vi "04Foot.vi"() -> ()   [LabVIEW 2020]
uses:
  <vilib>/DAQmx/read.llb/DAQmx Read (Digital 1D U8 1Chan NSamp).vi
  <vilib>/Instr/_visa.llb/VISA Configure Serial Port (Serial Instr).vi
  <vilib>/Utility/file.llb/Read Delimited Spreadsheet (DBL).vi
  <vilib>/DAQmx/create/channels.llb/DAQmx Create Channel (DI-Digital Input).vi
  <vilib>/DAQmx/configure/timing.llb/DAQmx Timing (Change Detection).vi
  <vilib>/DAQmx/miscellaneous.llb/DAQmx Fill In Error Info.vi
panel:
  out "MPH READ 2":u8
  in  "Tab Control":enum32{"Page 1", "Page 2", "Page 3"}(tab)
  out "NEXT INC":dbl min=0.0 max=12.0 step=0.1 format="%.1f"
  out "INC":dbl min=0.0 max=12.0 step=0.1 format="%.1f"
  out "NEXT DURATION":dbl format="%#.1f"
  out "NEXT MPH":dbl min=0.0 max=12.0 step=0.1 format="%.1f"
  out "Time Left":dbl format="%#.0f"
  out "ESTOP":bool
  in  "ESTOP RESUME":bool
  out "MPH":dbl min=0.0 max=12.0 step=0.1 format="%.1f"
  out "incline":dbl[](array[numeric])
  out "ESTOP2":bool
  out "Report Location":path
  in  "TestScript":path=path "C:/LabView Computer Backup SEAL2788/DonP_TRM500/FootTimeInc.txt"
  out "Waveform Graph":dbl[](graph)
  out "speed":dbl[](array[numeric])
  out "time":dbl[](array[numeric])
  out "dwell":dbl[](array[numeric])
  out "step":i32
  out "arraysize":i32
  out "x-y":u32
  out "appended path":path
  out "stopping":bool
  out "String":string
  in  "stop":bool
  out "MPH READ":u8
  in  "Serial Port":refnum<visa-resource-name>="COM8"
  in  "lines":tag="cDAQ1Mod1/port0/line0"
  out "Enum":T1(ring)
  out "FootPath":path
  out "Array":T2(array[cluster])
  out "size(s)":i32
  out "FootPathRef":refnum<file>
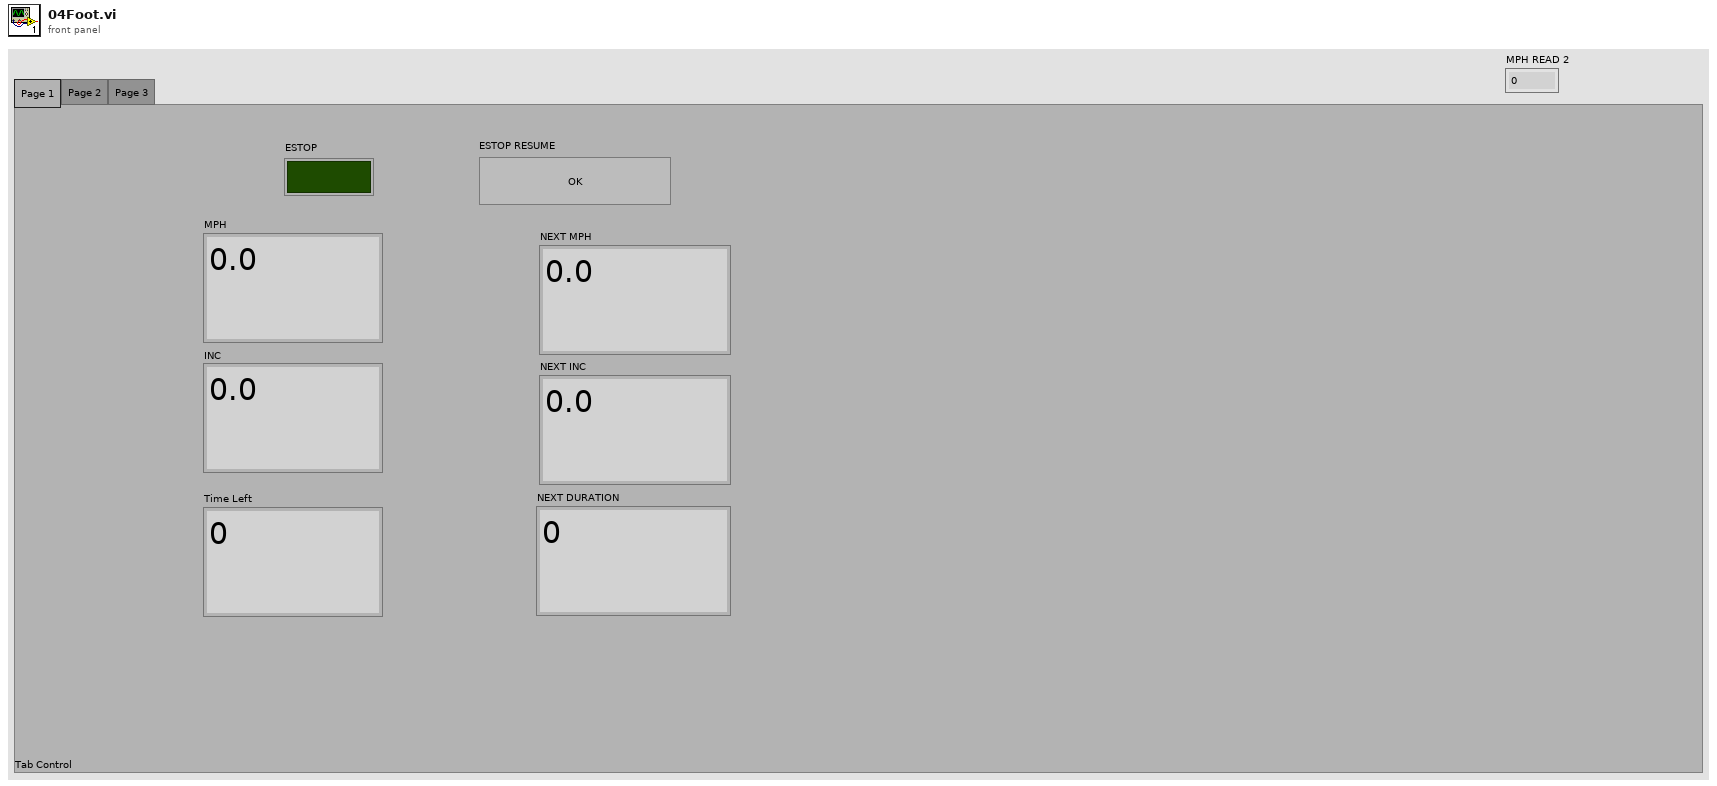
[diagram p1: front panel]
types:
  T1 = enum16{"Initialize", "SetMPH", "GetData", "CheckTiming", "CompressWave", "StartDAQ", "StopDAQ", "Dwell", "WaitforMPH", "ESTOP Wait", "ESTOP Resume"}
  T2 = cluster{"Trigger Time":timestamp, "MPH":dbl, "INC":dbl}[]
  T3 = cluster{"seconds since 1Jan1904":timestamp, "MPH":dbl, "INC":dbl}[]
  T4 = cluster{"Time":timestamp, "MPH":dbl, "INC":dbl}[]
  T5 = enum16{"Initialize", "SetMPH", "GetData", "CheckTiming", "CompressWave", "StartDAQ"}
  T6 = enum16{"Initialize", "SetMPH", "GetData", "CheckTiming", "CompressWave", "StartDAQ", "StopDAQ"}
  T7 = enum16{"Initialize", "SetMPH", "GetData", "CheckTiming", "CompressWave", "StartDAQ", "StopDAQ", "Dwell", "WaitforMPH"}
  T8 = cluster{"seconds since 1Jan1904":timestamp, "MPH":dbl, "INC":dbl}
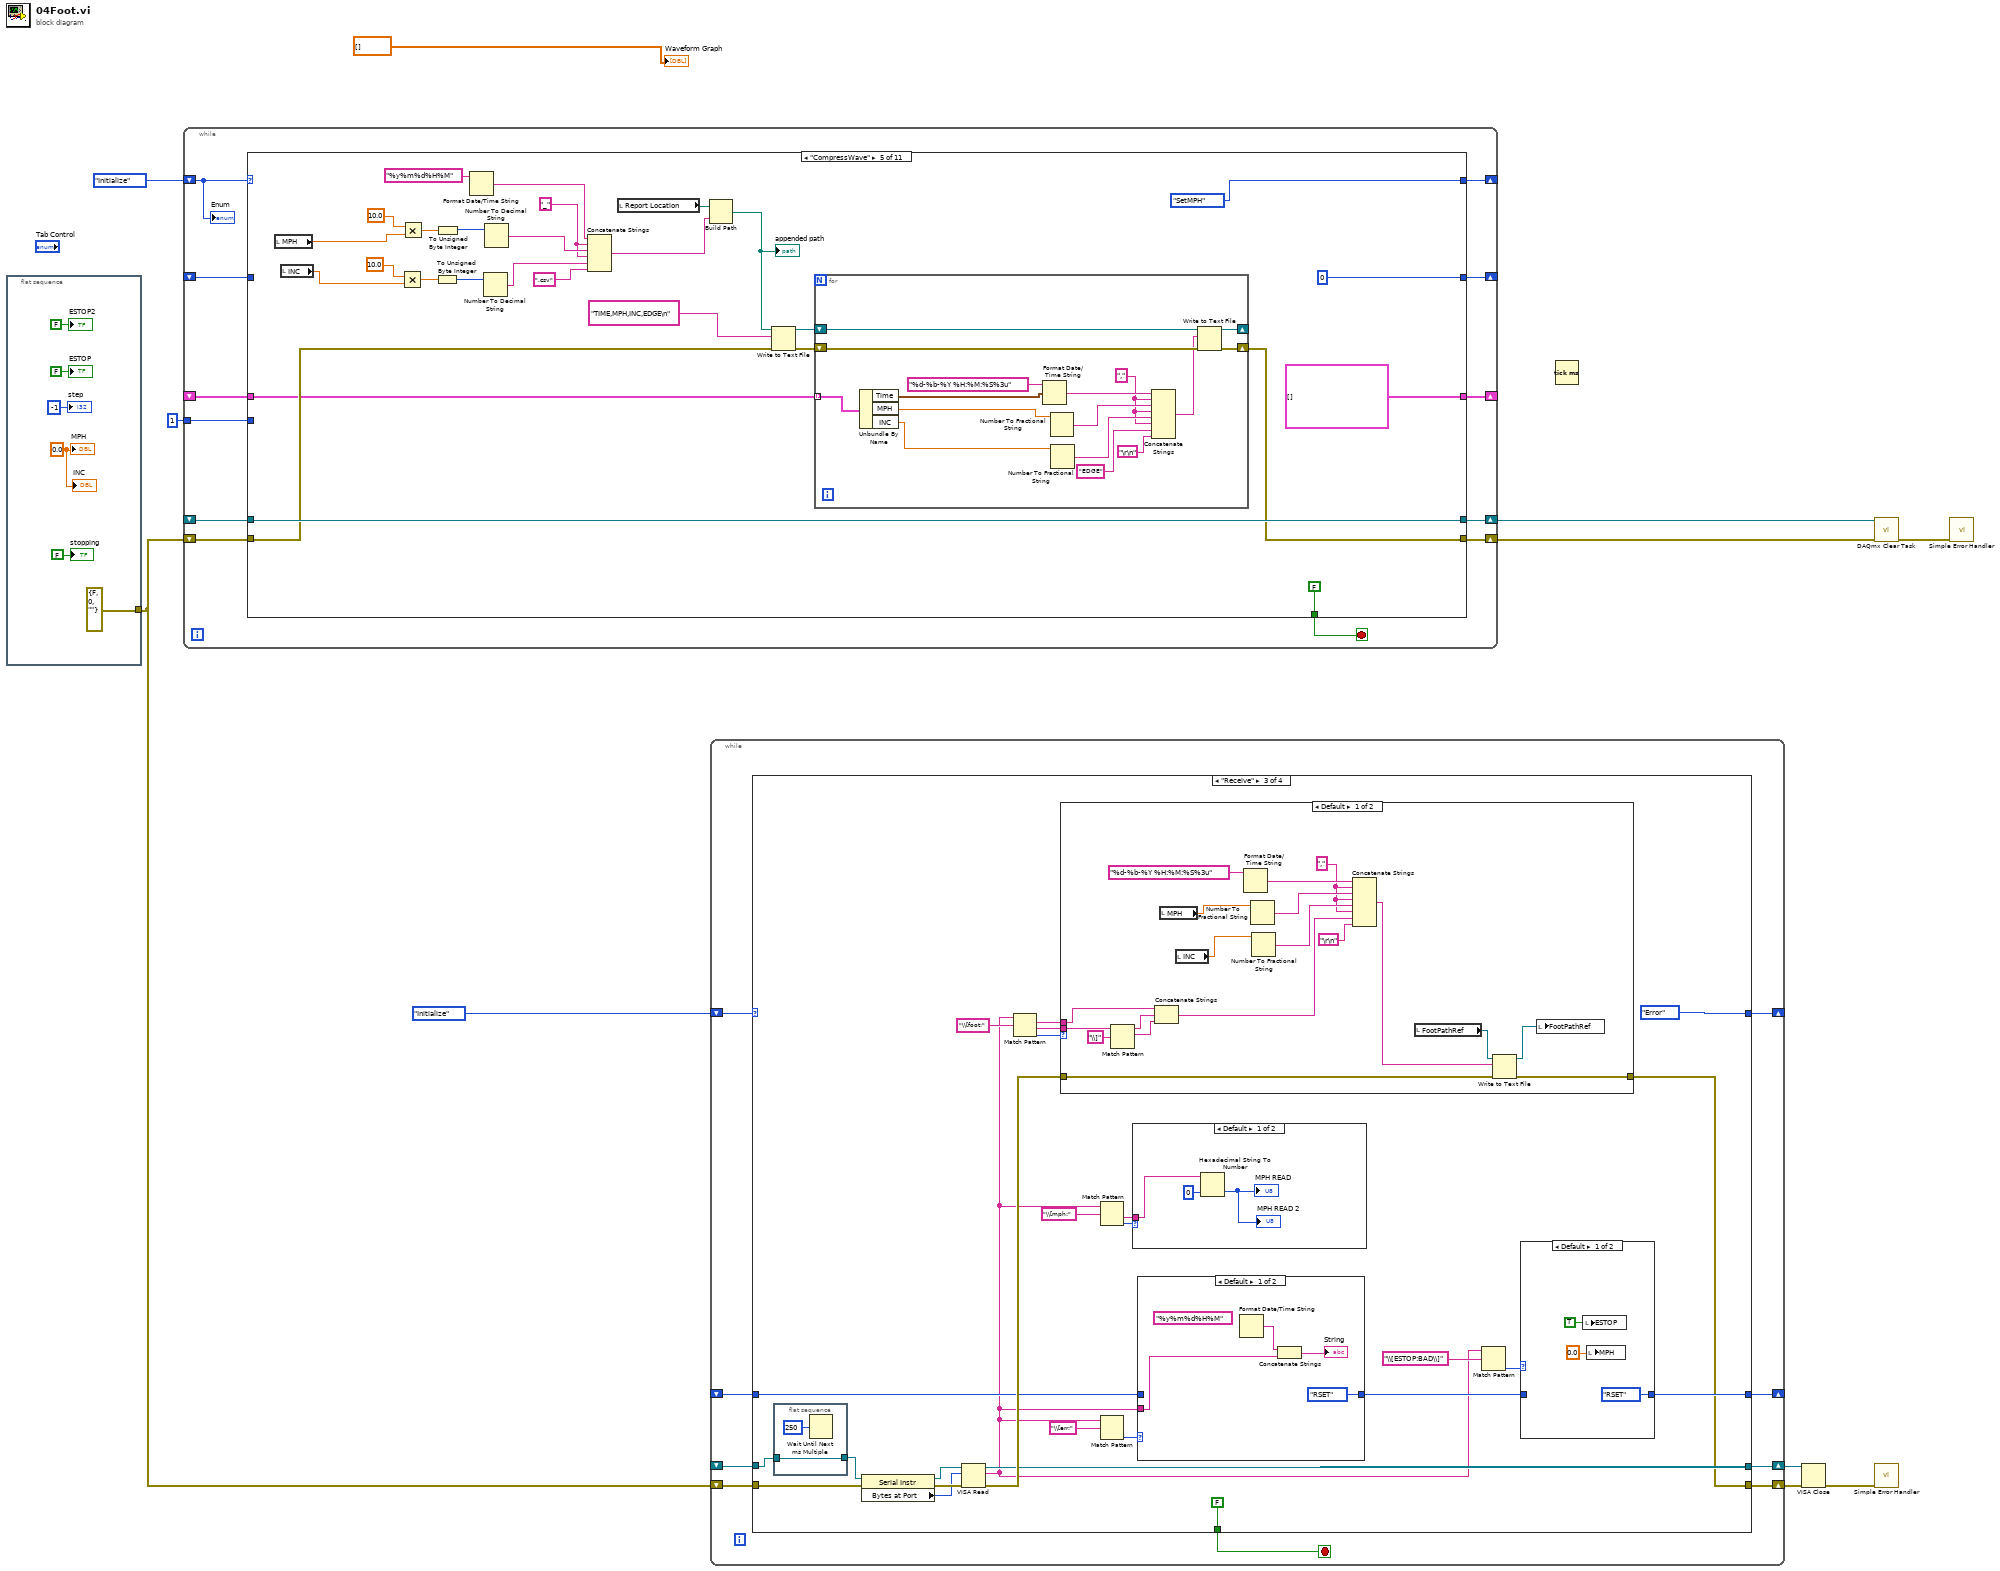
[diagram p0: block diagram]
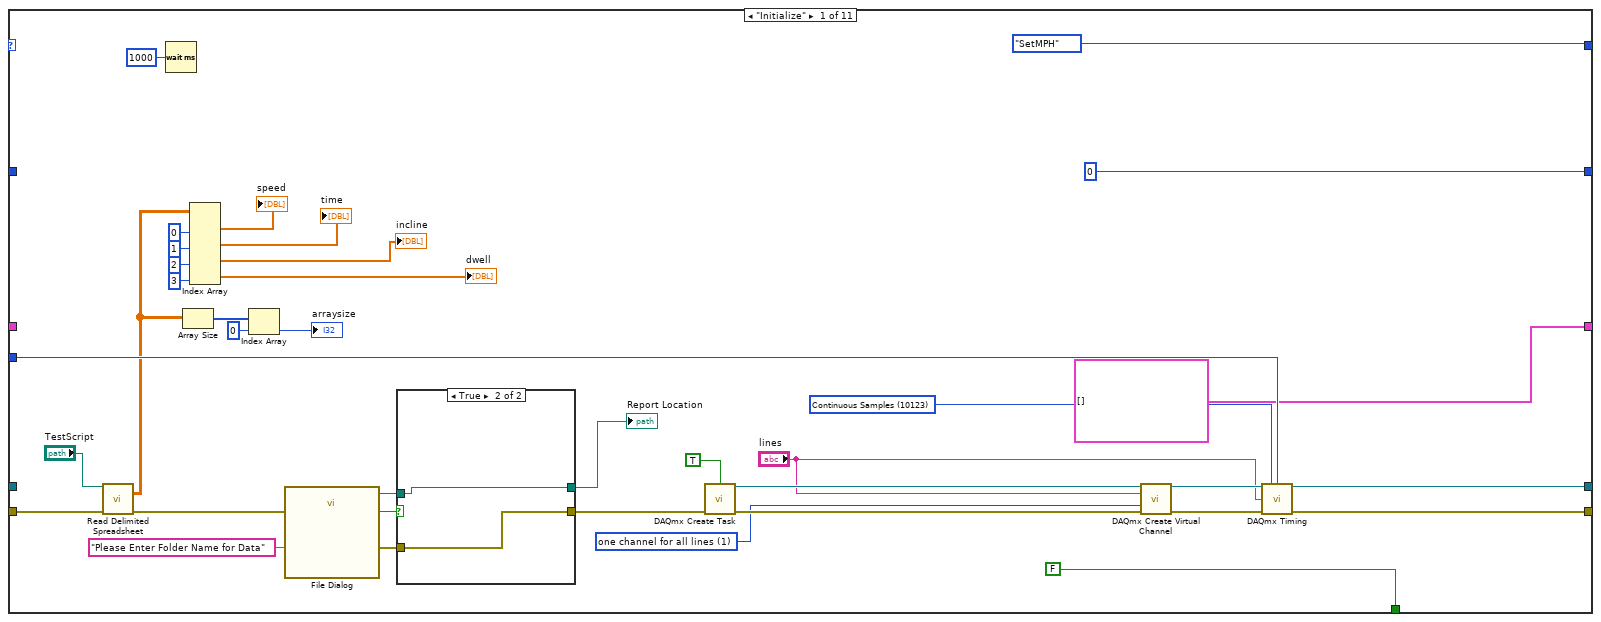
[diagram p2: hidden frame]
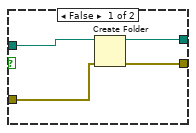
[diagram p3: hidden frame]
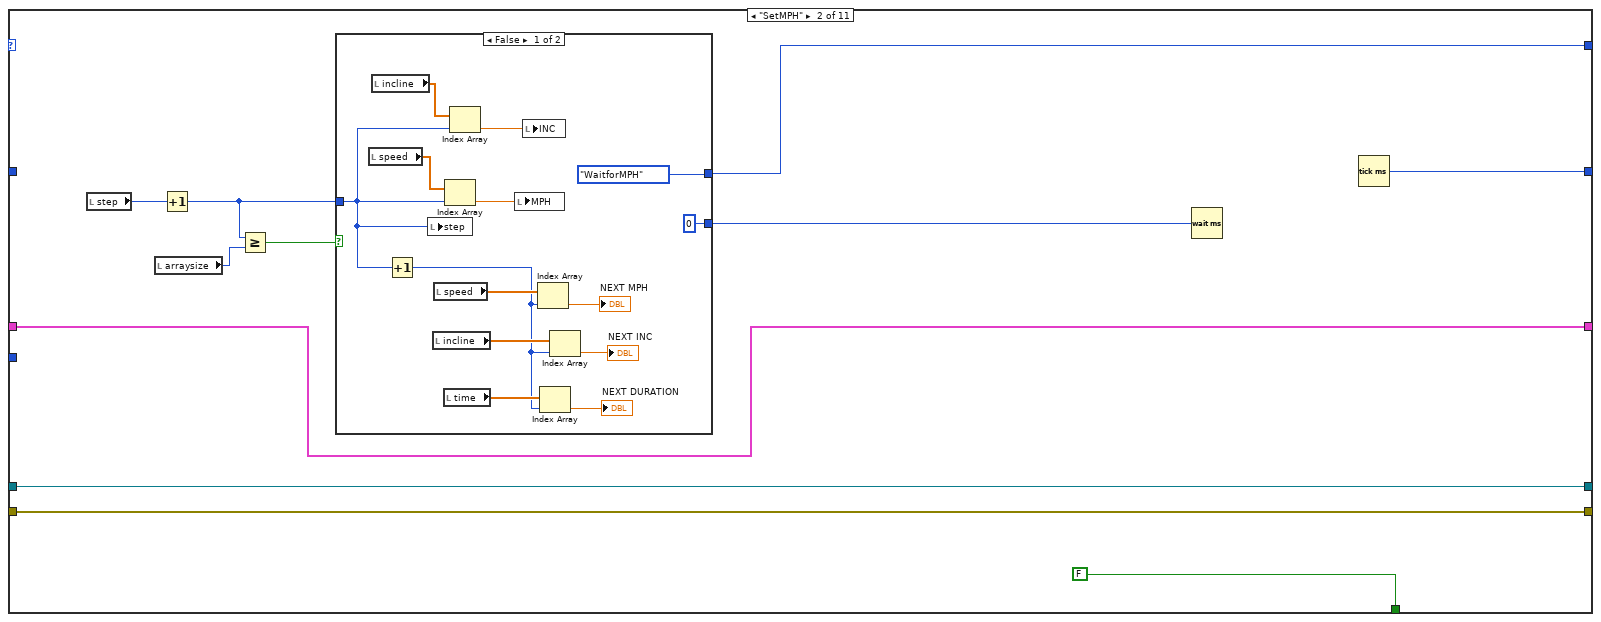
[diagram p4: hidden frame]
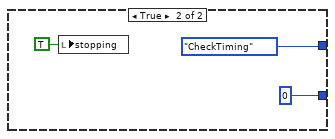
[diagram p5: hidden frame]
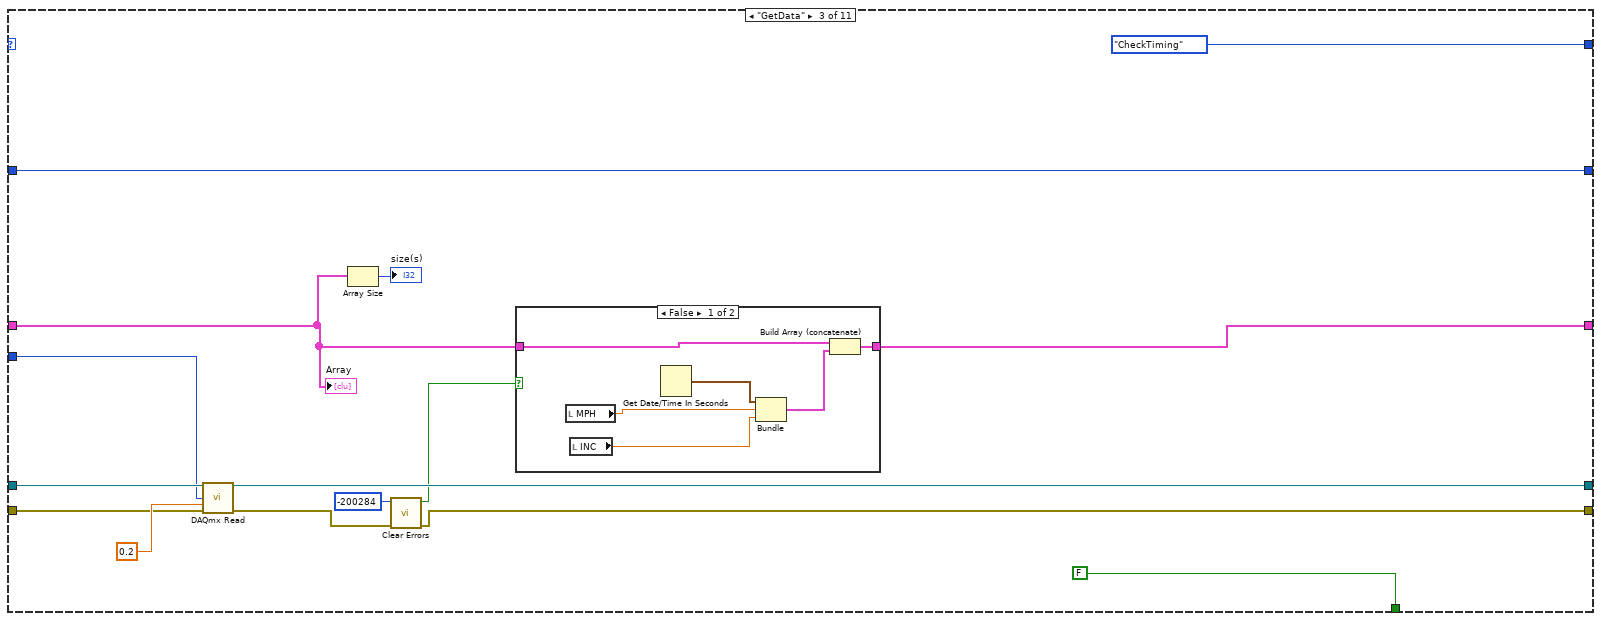
[diagram p6: hidden frame]
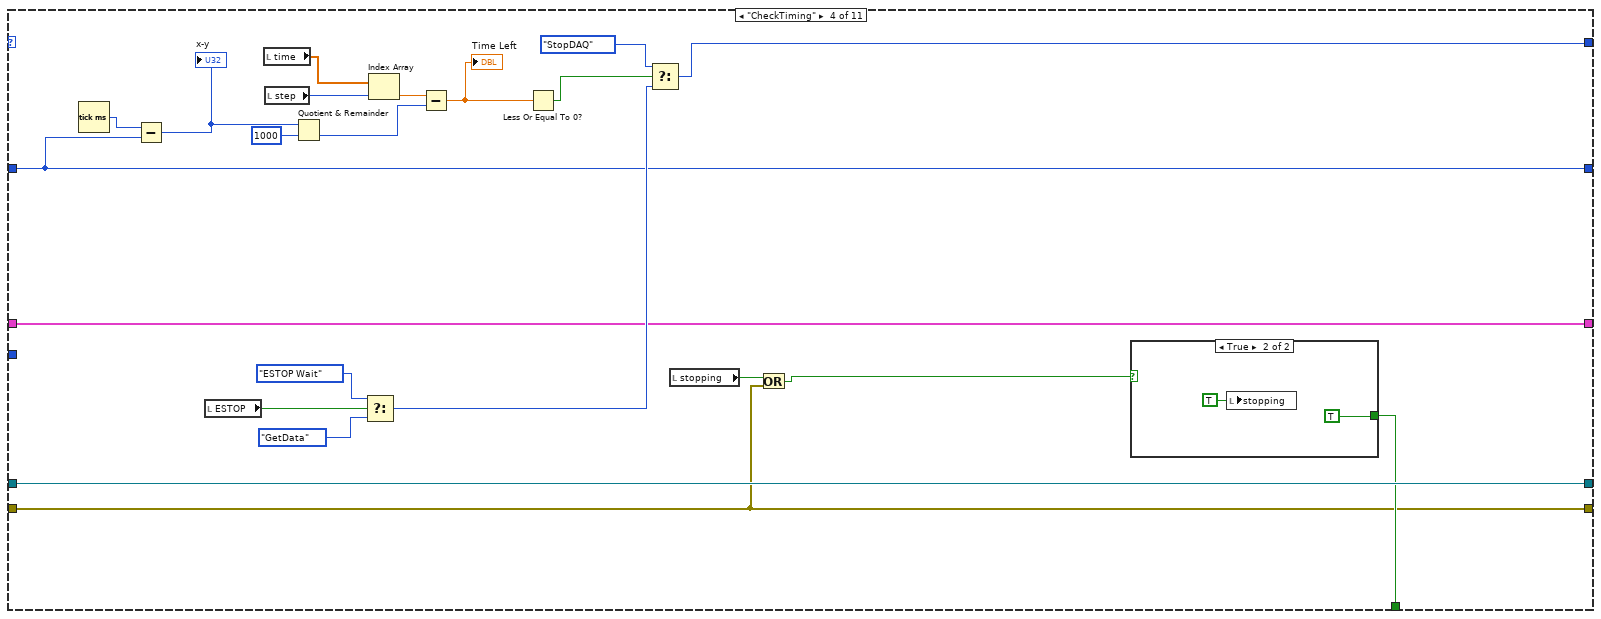
[diagram p8: hidden frame]
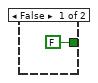
[diagram p9: hidden frame]
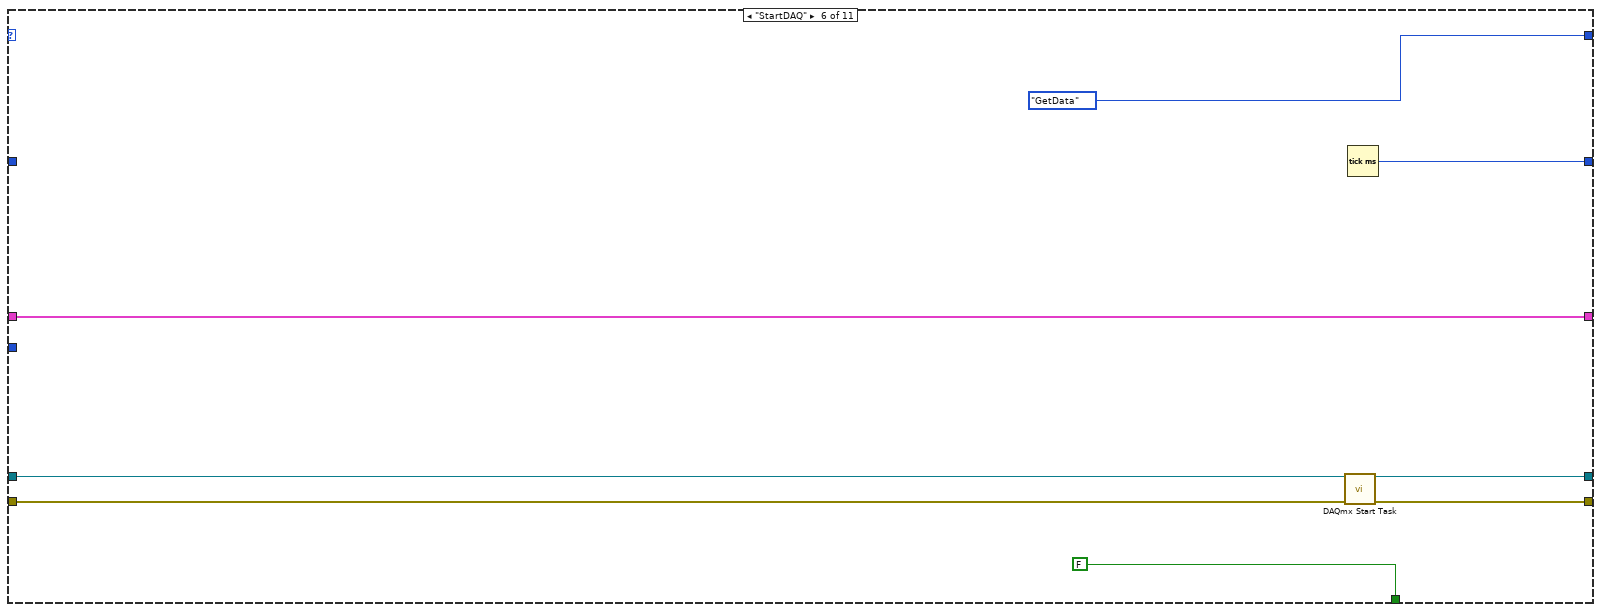
[diagram p10: hidden frame]
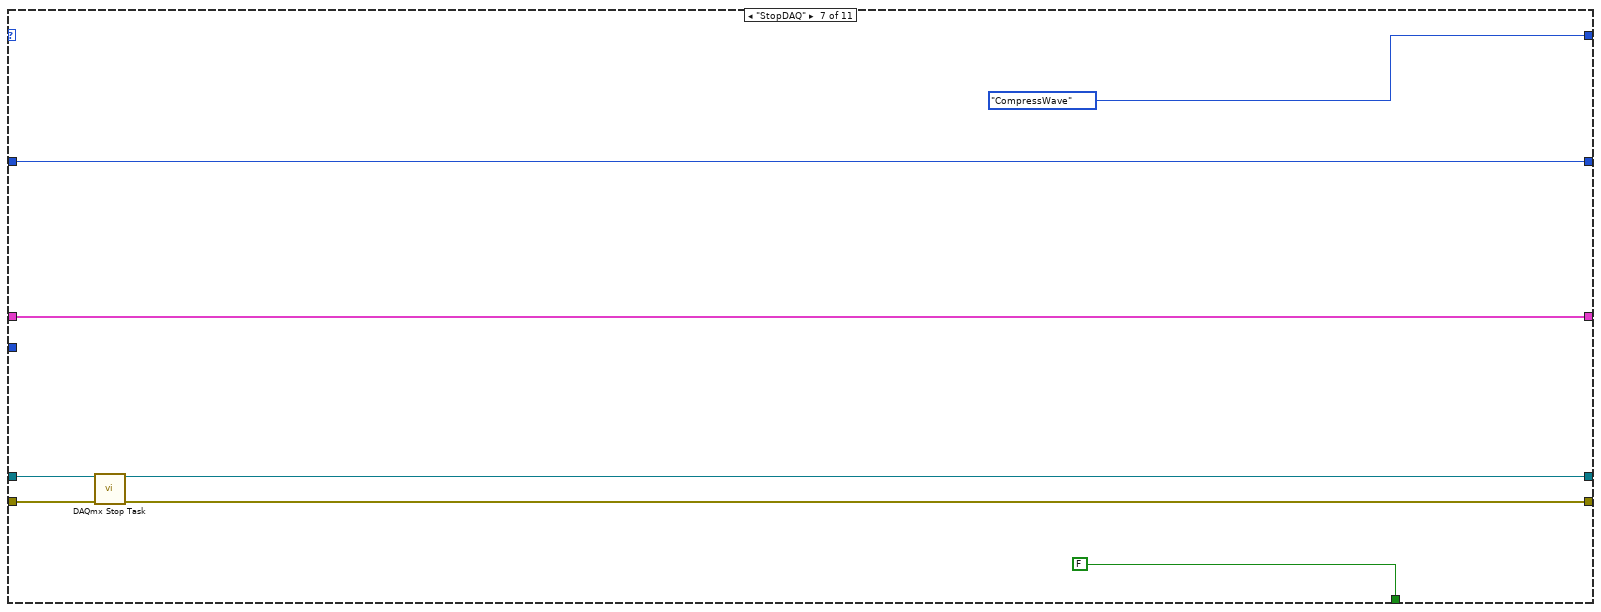
[diagram p11: hidden frame]
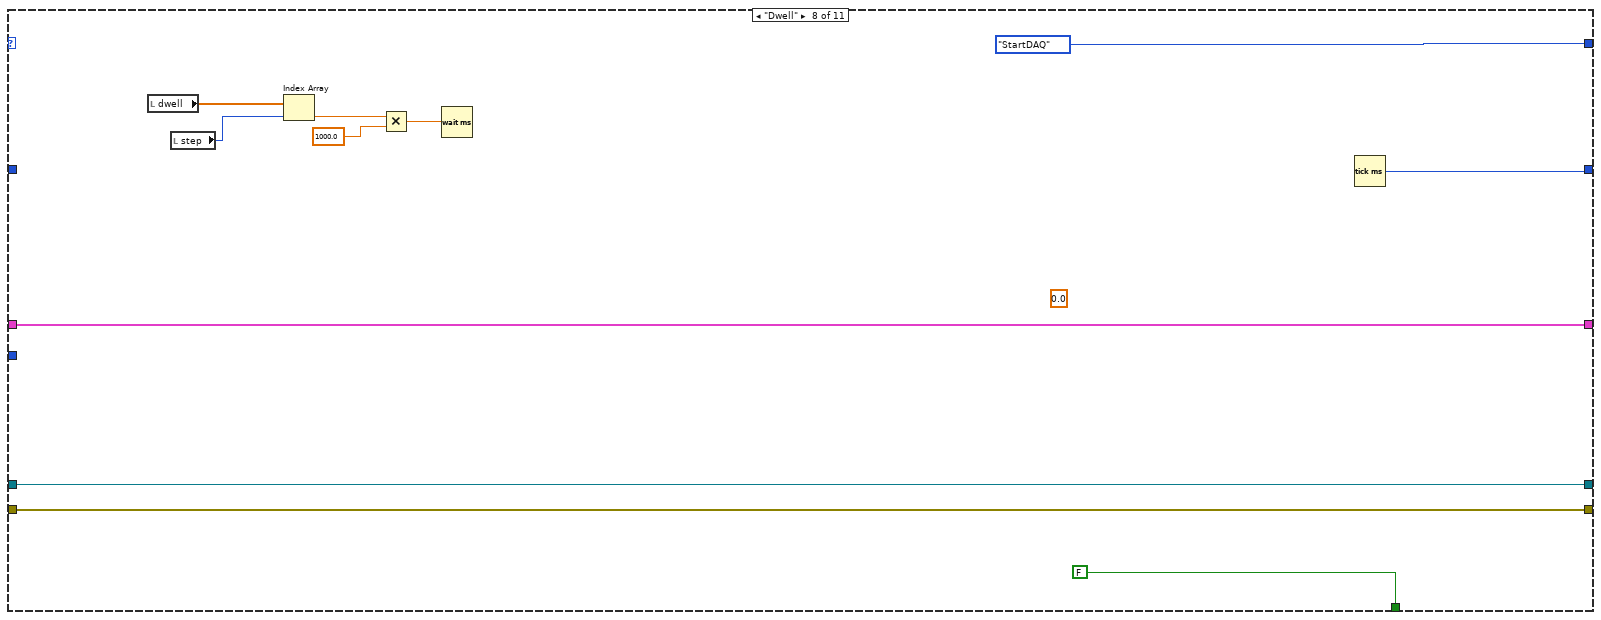
[diagram p12: hidden frame]
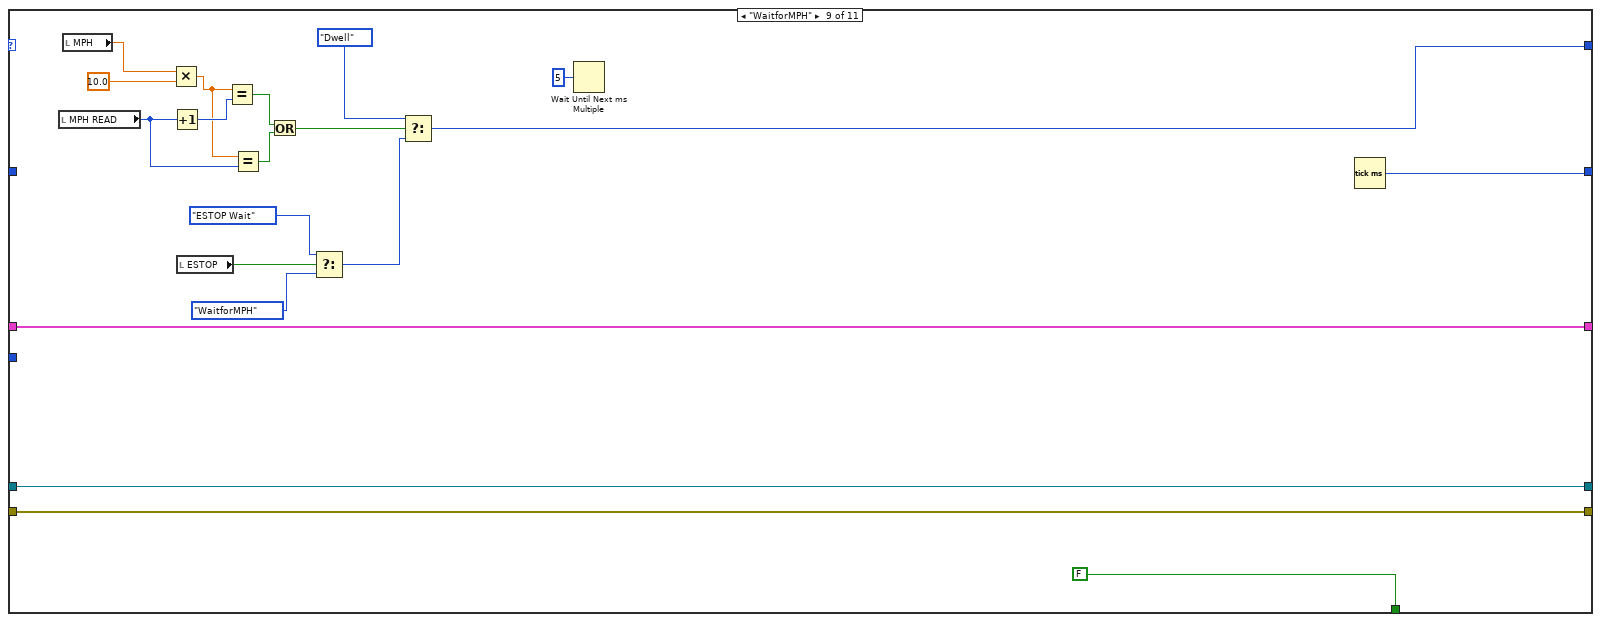
[diagram p13: hidden frame]
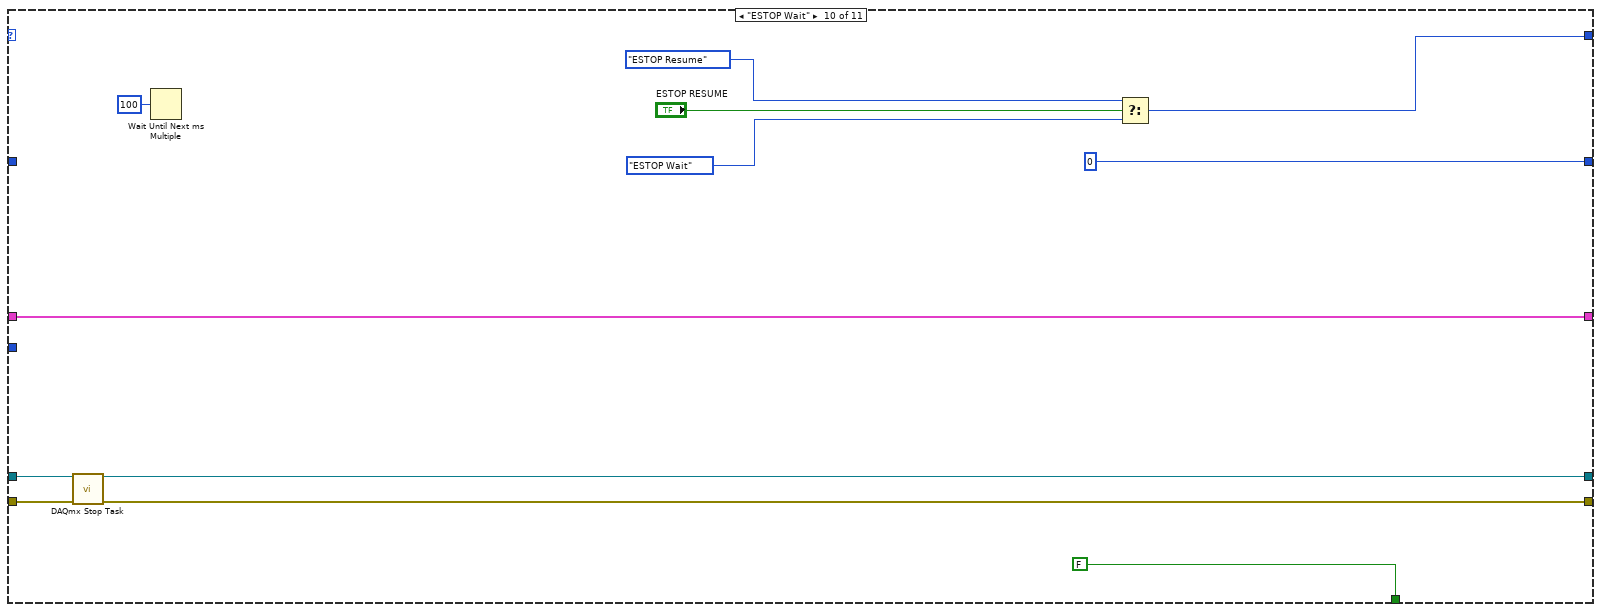
[diagram p14: hidden frame]
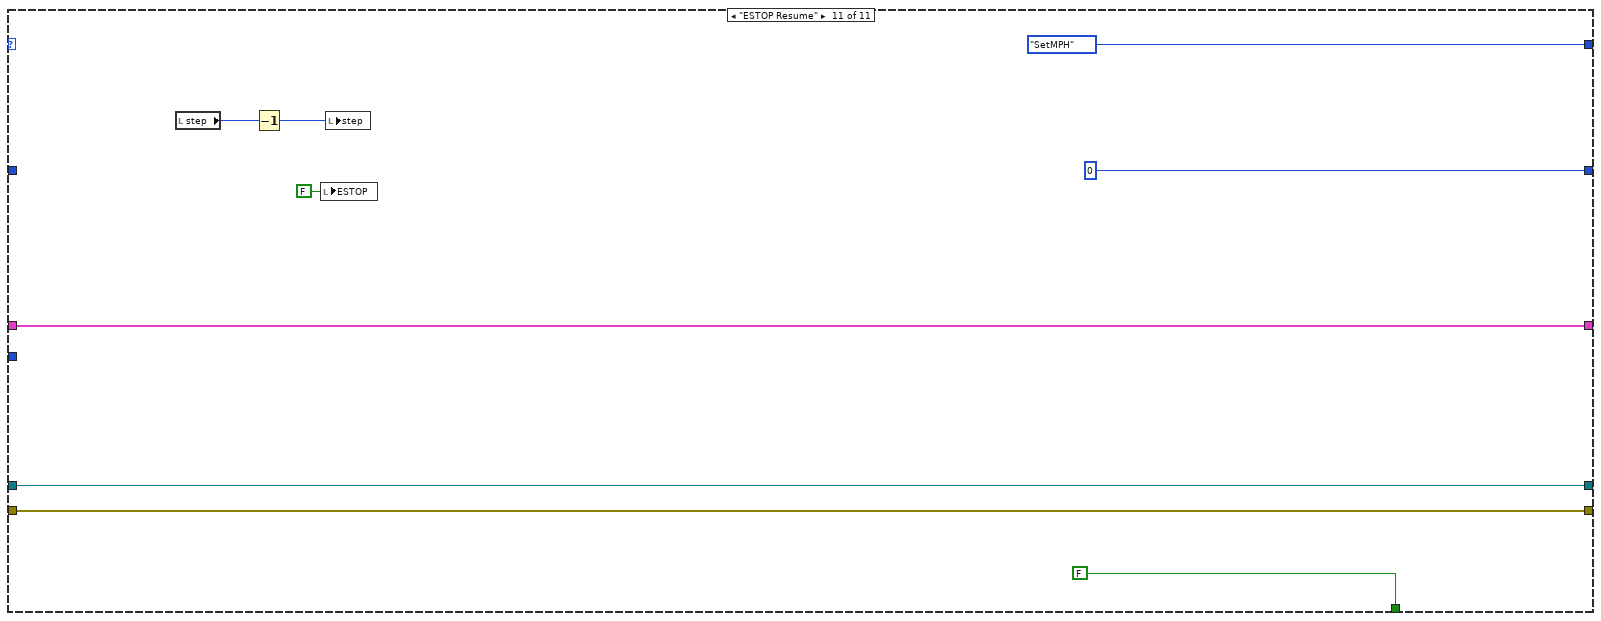
[diagram p15: hidden frame]
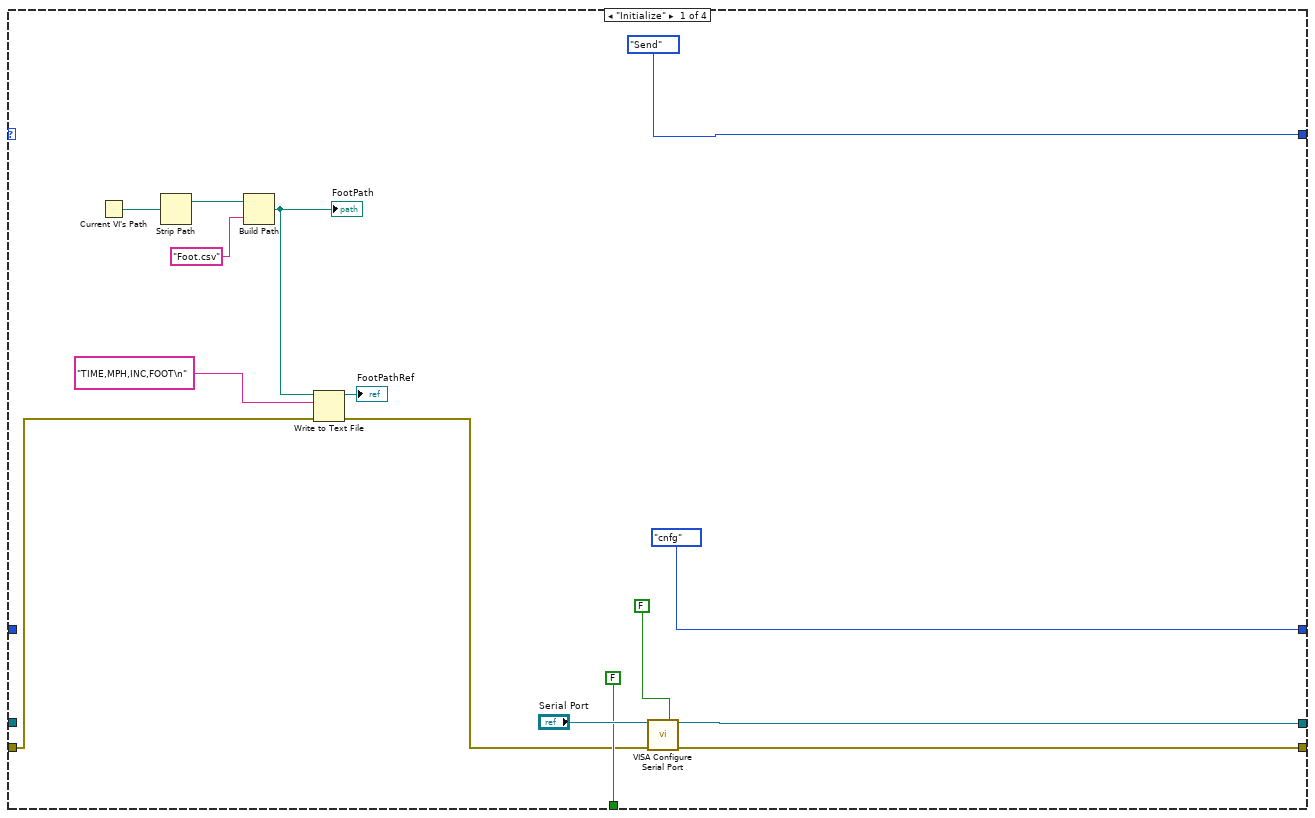
[diagram p16: hidden frame]
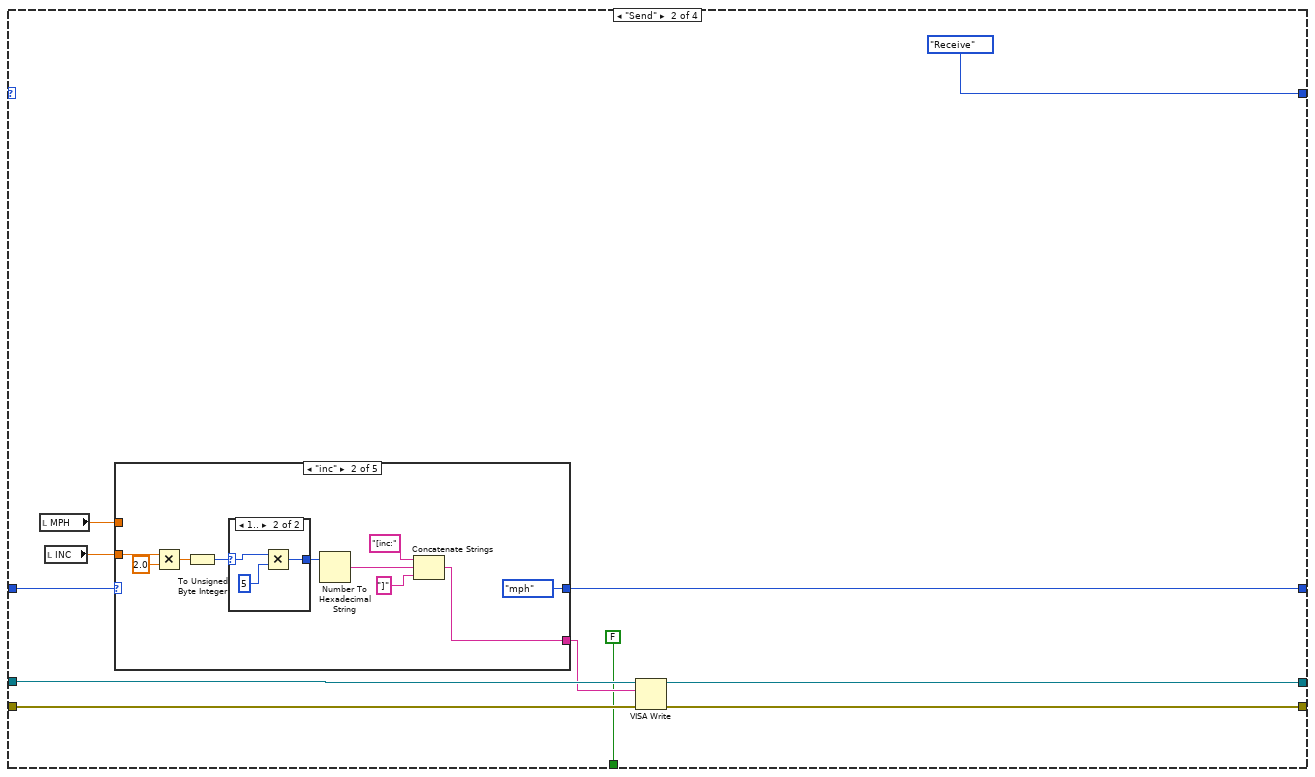
[diagram p17: hidden frame]
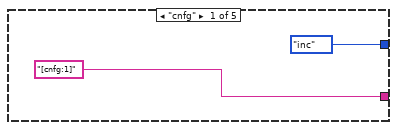
[diagram p18: hidden frame]
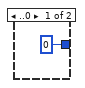
[diagram p19: hidden frame]
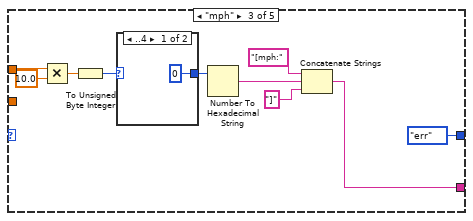
[diagram p20: hidden frame]
diagram:
  n1 = flat-sequence {
    tunnel: [errorcluster {"status"=FALSE, "code"=0, "source"=""} ("error constant")] -> w3
    frame #0 {
      w12 = 0.0 ("MPH")
      "stopping" <- FALSE ("stopping")
      "MPH" <- w12
      "step" <- -1 ("step")
      "ESTOP" <- FALSE ("ESTOP")
      "ESTOP2" <- FALSE ("ESTOP2")
      "INC" <- w12
    }
  }
  n2 = while {
    shift-right: [w29] -> _
    shift-left: T1."Initialize" -> [w20]
    shift-right: [w27] -> w5
    shift-left: _ -> [w25]
    shift-right: [w26] -> w6
    shift-left: w3 -> [w24]
    shift-right: [w23] -> _
    shift-left: _ -> [w22]
    tunnel: 1 ("samples per channel") -> [w21]
    shift-right: [w18] -> _
    shift-left: _ -> [w19]
    stop <- w28 stop-if-true
    n3 = case shown="\"CompressWave\"" w20 {
      tunnel: [T1."SetMPH" w79 T1."CheckTiming" ("f") w139 T1."SetMPH" T5."GetData" T6."CompressWave" T7."StartDAQ" w231 w245 T1."SetMPH" ("f")] -> w29
      tunnel: [FALSE FALSE FALSE w143 FALSE FALSE FALSE FALSE FALSE FALSE FALSE] -> w28
      tunnel: [w35 w81 w107 w144 w166 w196 w204 w217 w237 w241 w254] -> w27
      tunnel: [w36 w80 w106 w140 w148 w197 w203 w216 w236 w240 w255] -> w26
      tunnel: w25 -> [_ w81 w110 w144 w166 w195 w206 w217 w237 w243 w254]
      tunnel: w24 -> [w60 w80 w109 w140 w152 w194 w205 w216 w236 w242 w255]
      tunnel: [u32 0 w73 w114 w127 u32 0 w192 w201 w218 w238 u32 0 ("millisecond timer value") u32 0 ("millisecond timer value")] -> w23
      tunnel: w22 -> [_ _ w114 w127 _ _ w201 _ _ _ _]
      tunnel: w21 -> [w57 _ w108 _ _ _ _ _ _ _ _]
      tunnel: w19 -> [_ w74 w102 w126 w151 w193 w200 w208 w219 w239 w251]
      tunnel: [T3 [] w74 w105 w126 T4 [] w193 w200 w208 w219 w239 w251] -> w18
      frame "Initialize" {
        w56 = 10123 items=["Finite Samples"=10178, "Continuous Samples"=10123, "Hardware Timed Single Point"=12522] ("sample mode")
        w64 = 1 items=["one channel for each line", "one channel for all lines"] ("line grouping")
        n4 = call-poly <vilib>:"Read Delimited Spreadsheet.vi"("file path (dialog if empty)"="TestScript", "error in (no error)"=w60) -> ("all rows"=w47:dbl[][], "error out"=w45:errorcluster)  [unwired: 8 in, 4 out]
        n5 = Wait (ms)(milliseconds to wait=u32 1000) -> ()  [unwired: 1 out]
        n6 = Array Size(array=w47) -> (size(s)=w50:i32[])
        n7 = Index Array(array=w47, index (col) #1=0 ("disabled index (col)"), index (col) #2=1 ("index (col)"), index (col) #3=2 ("index (col)"), index (col) #4=3 ("index (col)")) -> (element #1=→"speed":dbl[], element #2=→"time":dbl[], element #3=→"incline":dbl[], element #4=→"dwell":dbl[])  [unwired: 4 in]
        n8 = Index Array(array=w50, index=0) -> (element=→"arraysize":i32)
        n9 = call "File Dialog"("prompt"="Please Enter Folder Name for Data", "error in"=w45) -> ("selected path"=w41:path, "exists"=w43:bool, "error out"=w42:errorcluster)  [unwired: 10 in, 1 out]
        n10 = case shown="True" w43 {
          tunnel: w42 -> [w70 w71]
          tunnel: w41 -> [w69 w72]
          tunnel: [w68 w71] -> w40
          tunnel: [w67 w72] -> w39
          frame False {
            n11 = Create Folder(path (use dialog)=w69, error in=w70) -> (created path=w67:path, error out=w68:errorcluster)  [unwired: 1 in, 1 out]
          }
          frame True {
          }
        }
        "Report Location" <- w39
        n12 = call <vilib>:"DAQmx Create Task.vi"("auto cleanup"=TRUE, "error in"=w40) -> ("task out"=w66:refnum<k21>, "error out"=w65:errorcluster)  [unwired: 12 in]
        n13 = call-poly <vilib>:"DAQmx Create Virtual Channel.vi"("task in"=w66, "lines"="lines", "line grouping"=w64, "error in"=w65) -> ("task out"=w58:refnum<k21>, "error out"=w59:errorcluster)  [unwired: 10 in]
        n14 = call-poly <vilib>:"DAQmx Timing.vi"("task/channels in"=w58, "sample mode"=w56, "samples per channel"=w57, "rising edge physical channels"="lines", "error in"=w59) -> ("task out"=w35:refnum<k21>, "error out"=w36:errorcluster)  [unwired: 9 in]
      }
      frame "SetMPH" {
        n15 = local read "step"() -> (w76:i32)
        n16 = local read "arraysize"() -> (w78:i32)
        n17 = Increment(x=w76) -> (x+1=w75:i32)
        n18 = Greater Or Equal?(x=w75, y=w78) -> (x >= y?=w77:bool)
        n19 = case shown="False" w77 {
          tunnel: [u32 0 ("milliseconds to wait") u32 0 ("milliseconds to wait")] -> w82
          tunnel: [T1."WaitforMPH" T1."CheckTiming"] -> w79
          tunnel: w75 -> [w86 _]
          frame False {
            n20 = local read "speed"() -> (w96:dbl[])
            n21 = local read "incline"() -> (w87:dbl[])
            n22 = Increment(x=w86) -> (x+1=w88:i32)
            n23 = local write "step"(w86) -> ()
            n24 = local read "incline"() -> (w89:dbl[])
            n25 = local read "speed"() -> (w94:dbl[])
            n26 = local read "time"() -> (w91:dbl[])
            n27 = Index Array(array=w96, index=w86) -> (element=w95:dbl)
            n28 = Index Array(array=w87, index=w86) -> (element=w85:dbl)
            n29 = local write "MPH"(w95) -> ()
            n30 = local write "INC"(w85) -> ()
            n31 = Index Array(array=w94, index=w88) -> (element=→"NEXT MPH":dbl)
            n32 = Index Array(array=w91, index=w88) -> (element=→"NEXT DURATION":dbl)
            n33 = Index Array(array=w89, index=w88) -> (element=→"NEXT INC":dbl)
          }
          frame True {
            n34 = local write "stopping"(TRUE ("stopping")) -> ()
          }
        }
        n35 = Wait (ms)(milliseconds to wait=w82) -> ()  [unwired: 1 out]
        n36 = Tick Count (ms)() -> (millisecond timer value=w73:u32)
      }
      frame "GetData" {
        n37 = call-poly <vilib>:"DAQmx Read.vi"("task/channels in"=w110, "number of samples per channel"=w108, "timeout"=0.2, "error in"=w109) -> ("task out"=w107:refnum<k21>, "error out"=w111:errorcluster)  [unwired: 9 in, 1 out]
        n38 = Array Size(array=w102) -> (size(s)=→"size(s)":i32)
        n39 = call <vilib>:"Clear Errors.vi"("error in (no error)"=w111, "specific error code to clear (0: all)"=-200284) -> ("error out"=w106:errorcluster, "specific error cleared?"=w103:bool)  [unwired: 4 in]
        n40 = case shown="False" w103 {
          tunnel: [w121 w122] -> w105
          tunnel: w102 -> [w120 w122]
          frame False {
            n41 = local read "MPH"() -> (w117:dbl)
            n42 = local read "INC"() -> (w116:dbl)
            n43 = Get Date/Time In Seconds() -> (seconds since 1Jan1904=w119:timestamp)
            n44 = Bundle("seconds since 1Jan1904"=w119, "MPH"=w117, "INC"=w116) -> (w118:T8)  [unwired: 1 in]
            n45 = Build Array (concatenate)(w120, w118) -> (w121:T3)
          }
          frame True {
          }
        }
        "Array" <- w102
      }
      frame "CheckTiming" {
        n46 = Tick Count (ms)() -> (millisecond timer value=w128:u32)
        n47 = Subtract(x=w128, y=w127) -> (x-y=w125:u32)
        "x-y" <- w125
        n48 = local read "ESTOP"() -> (w134:bool)
        n49 = local read "time"() -> (w138:dbl[])
        n50 = local read "step"() -> (w137:i32)
        n51 = Quotient & Remainder(x=w125, y=u32 1000) -> (floor(x/y)=w123:u32)  [unwired: 1 out]
        n52 = Select(t=T1."ESTOP Wait", s=w134, f=T1."GetData") -> (s? t:f=w132:T1)
        n53 = Index Array(array=w138, index=w137) -> (element=w131:dbl)
        n54 = Subtract(x=w131, y=w123) -> (x-y=w130:dbl)
        "Time Left" <- w130
        n55 = Less Or Equal To 0?(x=w130) -> (x <= 0?=w129:bool)
        n56 = Select(t=T1."StopDAQ", s=w129, f=w132) -> (s? t:f=w139:T1)
        n57 = local read "stopping"() -> (w142:bool)
        n58 = Or(x=w142, y=w140) -> (x .or. y?=w141:bool)
        n59 = case shown="True" w141 {
          tunnel: [FALSE TRUE] -> w143
          frame False {
          }
          frame True {
            n60 = local write "stopping"(TRUE ("stopping")) -> ()
          }
        }
      }
      frame "CompressWave" {
        w160 = "_" ("string")
        n61 = local read "MPH"() -> (w167:dbl)
        n62 = local read "INC"() -> (w156:dbl)
        n63 = Multiply(x=10.0, y=w156) -> (x*y=w158:dbl)
        n64 = Multiply(x=10.0, y=w167) -> (x*y=w170:dbl)
        n65 = To Unsigned Byte Integer(number=w158) -> (unsigned 8bit integer=w157:u8)
        n66 = To Unsigned Byte Integer(number=w170) -> (unsigned 8bit integer=w169:u8)
        n67 = Format Date/Time String(time format string (%c)="%y%m%d%H%M") -> (date/time string=w163:string)  [unwired: 2 in]
        n68 = Number To Decimal String(number=w157) -> (decimal integer string=w155:string)  [unwired: 1 in]
        n69 = Number To Decimal String(number=w169) -> (decimal integer string=w168:string)  [unwired: 1 in]
        n70 = Concatenate Strings(w163, w160, w168, w160, w155, ".csv" ("string")) -> (w172:string)
        n71 = local read "Report Location"() -> (w165:path)
        n72 = Build Path(base path=w165, name or relative path=w172) -> (appended path=w153:path)
        "appended path" <- w153
        n73 = Write to Text File(file (use dialog)=w153, text="TIME,MPH,INC,EDGE\n", error in=w152) -> (refnum out=w150:refnum<file>, error out=w149:errorcluster)  [unwired: 1 in, 1 out]
        n74 = for {
          tunnel: w151 -> [w191] mode=indexing
          shift-right: [w177] -> _
          shift-left: w150 -> [w180]
          shift-right: [w176] -> w148
          shift-left: w149 -> [w179]
          w185 = ","
          n75 = Unbundle By Name(w191) -> ("Time"=w183:timestamp, "MPH"=w182:dbl, "INC"=w181:dbl)
          n76 = Format Date/Time String(time format string (%c)="%d-%b-%Y %H:%M:%S%3u", seconds (now)=w183) -> (date/time string=w189:string)  [unwired: 1 in]
          n77 = Number To Fractional String(number=w182) -> (F-format string=w188:string)  [unwired: 3 in]
          n78 = Number To Fractional String(number=w181) -> (F-format string=w187:string)  [unwired: 3 in]
          n79 = Concatenate Strings(w189, w185, w188, w185, w187, w185, "EDGE", "\r\n") -> (w178:string)
          n80 = Write to Text File(file (use dialog)=w180, text=w178, error in=w179) -> (refnum out=w177:refnum<file>, error out=w176:errorcluster)  [unwired: 1 in, 1 out]
        }
      }
      frame "StartDAQ" {
        n81 = call <vilib>:"DAQmx Start Task.vi"("task/channels in"=w195, "error in"=w194) -> ("task out"=w196:refnum<k21>, "error out"=w197:errorcluster)  [unwired: 12 in]
        n82 = Tick Count (ms)() -> (millisecond timer value=w192:u32)
      }
      frame "StopDAQ" {
        n83 = call <vilib>:"DAQmx Stop Task.vi"("task/channels in"=w206, "error in"=w205) -> ("task out"=w204:refnum<k21>, "error out"=w203:errorcluster)  [unwired: 12 in]
      }
      frame "Dwell" {
        (unwired) 0.0
        n84 = local read "dwell"() -> (w214:dbl[])
        n85 = local read "step"() -> (w213:i32)
        n86 = Index Array(array=w214, index=w213) -> (element=w212:dbl)
        n87 = Multiply(x=w212, y=1000.0) -> (x*y=w210:dbl)
        n88 = Wait (ms)(milliseconds to wait=w210) -> ()  [unwired: 1 out]
        n89 = Tick Count (ms)() -> (millisecond timer value=w218:u32)
      }
      frame "WaitforMPH" {
        n90 = local read "MPH READ"() -> (w223:u8)
        n91 = local read "MPH"() -> (w234:dbl)
        n92 = Multiply(x=w234, y=10.0) -> (x*y=w224:dbl)
        n93 = Increment(x=w223) -> (x+1=w232:u8)
        n94 = local read "ESTOP"() -> (w229:bool)
        n95 = Equal?(x=w224, y=w232) -> (x = y?=w221:bool)
        n96 = Equal?(x=w224, y=w223) -> (x = y?=w222:bool)
        n97 = Or(x=w221, y=w222) -> (x .or. y?=w220:bool)
        n98 = Select(t=T1."ESTOP Wait", s=w229, f=T1."WaitforMPH") -> (s? t:f=w226:T1)
        n99 = Select(t=T1."Dwell", s=w220, f=w226) -> (s? t:f=w231:T1)
        n100 = Wait Until Next ms Multiple(millisecond multiple=u32 5) -> ()  [unwired: 1 out]
        n101 = Tick Count (ms)() -> (millisecond timer value=w238:u32)
      }
      frame "ESTOP Wait" {
        n102 = call <vilib>:"DAQmx Stop Task.vi"("task/channels in"=w243, "error in"=w242) -> ("task out"=w241:refnum<k21>, "error out"=w240:errorcluster)  [unwired: 12 in]
        n103 = Wait Until Next ms Multiple(millisecond multiple=u32 100) -> ()  [unwired: 1 out]
        n104 = Select(t=T1."ESTOP Resume", s="ESTOP RESUME", f=T1."ESTOP Wait") -> (s? t:f=w245:T1)
      }
      frame "ESTOP Resume" {
        n105 = local read "step"() -> (w259:i32)
        n106 = Decrement(x=w259) -> (x-1=w258:i32)
        n107 = local write "ESTOP"(FALSE ("ESTOP")) -> ()
        n108 = local write "step"(w258) -> ()
      }
    }
    "Enum" <- w20
  }
  n109 = while {
    shift-right: [w264] -> w9
    shift-left: w3 -> [w268]
    shift-right: [w265] -> w10
    shift-left: _ -> [w267]
    shift-right: [w263] -> _
    shift-left: enum16{"Initialize", "Send", "Receive", "Error"}."Initialize" -> [w266]
    shift-right: [w262] -> _
    shift-left: _ -> [w261]
    stop <- w260 stop-if-true
    n110 = case shown="\"Receive\"" w266 {
      tunnel: w268 -> [w271 w292 w347 w388]
      tunnel: w267 -> [_ w291 w346 w392]
      tunnel: [w281 w294 w345 w392] -> w265
      tunnel: [w280 w293 w327 w388] -> w264
      tunnel: [enum16{"Initialize", "Send", "Receive", "Error"}."Send" enum16{"Initialize", "Send", "Receive", "Error"}."Receive" enum16{"Initialize", "Send", "Receive", "Error"}."Error" enum16{"Initialize", "Send", "Receive", "Error"}."Send"] -> w263
      tunnel: [enum16{"cnfg", "inc", "mph", "err", "RSET"}."cnfg" w288 w335 w393] -> w262
      tunnel: w261 -> [_ w289 w340 w393]
      tunnel: [FALSE FALSE FALSE w387] -> w260
      frame "Initialize" {
        n111 = Current VI's Path() -> (path=w276:path)
        n112 = Strip Path(path=w276) -> (stripped path=w275:path)  [unwired: 1 out]
        n113 = Build Path(base path=w275, name or relative path="Foot.csv") -> (appended path=w272:path)
        "FootPath" <- w272
        n114 = Write to Text File(file (use dialog)=w272, text="TIME,MPH,INC,FOOT\n", error in=w271) -> (refnum out=→"FootPathRef":refnum<file>, error out=w270:errorcluster)  [unwired: 1 in, 1 out]
        n115 = call-poly "VISA Configure Serial Port"("VISA resource name"="Serial Port", "Enable Termination\nChar (T)"=FALSE ("Enable Termination\nChar (T)"), "error in (no error)"=w270) -> ("VISA resource name out"=w281:refnum<visa-resource-name>, "error out"=w280:errorcluster)  [unwired: 11 in]
      }
      frame "Send" {
        n116 = local read "MPH"() -> (w285:dbl)
        n117 = local read "INC"() -> (w284:dbl)
        n118 = case shown="\"inc\"" w289 {
          tunnel: ["[cnfg:1]" w297 w311 "[err]" "[RSET]"] -> w290
          tunnel: w285 -> [_ _ w320 _ _]
          tunnel: [enum16{"cnfg", "inc", "mph", "err", "RSET"}."inc" enum16{"cnfg", "inc", "mph", "err", "RSET"}."mph" enum16{"cnfg", "inc", "mph", "err", "RSET"}."err" enum16{"cnfg", "inc", "mph", "err", "RSET"}."cnfg" enum16{"cnfg", "inc", "mph", "err", "RSET"}."cnfg"] -> w288
          tunnel: w284 -> [_ w298 _ _ _]
          frame "cnfg" {
          }
          frame "inc" {
            n119 = Multiply(x=w298, y=2.0) -> (x*y=w301:dbl)
            n120 = To Unsigned Byte Integer(number=w301) -> (unsigned 8bit integer=w300:u8)
            n121 = case shown="1.." w300 {
              selector: w300 -> [_ w310]
              tunnel: [u8 0 w309] -> w299
              frame ..0 {
              }
              frame 1.. {
                n122 = Multiply(x=w310, y=u8 5) -> (x*y=w309:u8)
              }
            }
            n123 = Number To Hexadecimal String(2:w299) -> (0:w304:string)  [unwired: 1 in]
            n124 = Concatenate Strings("[inc:" ("string"), w304, "]" ("string")) -> (w297:string)
          }
          frame "mph" {
            n125 = Multiply(x=w320, y=10.0) -> (x*y=w314:dbl)
            n126 = To Unsigned Byte Integer(number=w314) -> (unsigned 8bit integer=w313:u8)
            n127 = case shown="..4" w313 {
              selector: w313 -> [_ w322]
              tunnel: [u8 0 w322] -> w312
              frame ..4 {
              }
              frame 5.. {
              }
            }
            n128 = Number To Hexadecimal String(2:w312) -> (0:w317:string)  [unwired: 1 in]
            n129 = Concatenate Strings("[mph:" ("string"), w317, "]" ("string")) -> (w311:string)
          }
          frame "err" {
          }
          frame "RSET" {
          }
        }
        n130 = VISA Write(VISA resource name=w291, write buffer=w290, error in (no error)=w292) -> (VISA resource name out=w294:refnum<visa-resource-name>, error out=w293:errorcluster)  [unwired: 1 out]
      }
      frame "Receive" {
        n131 = flat-sequence {
          tunnel: w346 -> [w385]
          tunnel: [w385] -> w351
          frame #0 {
            n132 = Wait Until Next ms Multiple(millisecond multiple=u32 250) -> ()  [unwired: 1 out]
          }
        }
        n133 = property class="Serial Instr"(reference=w351, error in=w347) -> (reference out=w349:refnum<visa-resource-name>, error out=w350:errorcluster, "Bytes at Port"=w348:u32)
        n134 = VISA Read(VISA resource name=w349, byte count=w348, error in (no error)=w350) -> (VISA resource name out=w345:refnum<visa-resource-name>, read buffer=w331:string, error out=w352:errorcluster)  [unwired: 1 out]
        n135 = Match Pattern(string=w331, regular expression="\\[foot:") -> (match substring=w329:string, after substring=w328:string, offset past match=w330:i32)  [unwired: 1 in, 1 out]
        n136 = case shown="Default" w330 {
          tunnel: w329 -> [w369 _]
          tunnel: w328 -> [w371 _]
          tunnel: w352 -> [w359 w372]
          tunnel: [w356 w372] -> w327
          frame Default {
            w361 = ","
            n137 = Match Pattern(string=w371, regular expression="\\]") -> (before substring=w368:string, match substring=w367:string)  [unwired: 1 in, 2 out]
            n138 = Concatenate Strings(w369, w368, w367) -> (w360:string)
            n139 = local read "MPH"() -> (w355:dbl)
            n140 = local read "INC"() -> (w354:dbl)
            n141 = Format Date/Time String(time format string (%c)="%d-%b-%Y %H:%M:%S%3u") -> (date/time string=w365:string)  [unwired: 2 in]
            n142 = Number To Fractional String(number=w355) -> (F-format string=w364:string)  [unwired: 3 in]
            n143 = Number To Fractional String(number=w354) -> (F-format string=w363:string)  [unwired: 3 in]
            n144 = Concatenate Strings(w365, w361, w364, w361, w363, w361, w360, "\r\n") -> (w357:string)
            n145 = local read "FootPathRef"() -> (w358:refnum<file>)
            n146 = Write to Text File(file (use dialog)=w358, text=w357, error in=w359) -> (refnum out=w353:refnum<file>, error out=w356:errorcluster)  [unwired: 1 in, 1 out]
            n147 = local write "FootPathRef"(w353) -> ()
          }
          frame -1 {
          }
        }
        n148 = Match Pattern(string=w331, regular expression="\\[mph:") -> (after substring=w337:string, offset past match=w338:i32)  [unwired: 1 in, 2 out]
        n149 = Match Pattern(string=w331, regular expression="\\[err:") -> (offset past match=w341:i32)  [unwired: 1 in, 3 out]
        n150 = case shown="Default" w338 {
          tunnel: w337 -> [w379 _]
          frame Default {
            n151 = Hexadecimal String To Number(string=w379, default (0uL)=u8 0 ("default (0 I32)")) -> (number=→"MPH READ" →"MPH READ 2":u8)  [unwired: 1 in, 1 out]
          }
          frame -1 {
          }
        }
        n152 = case shown="Default" w341 {
          tunnel: [enum16{"cnfg", "inc", "mph", "err", "RSET"}."RSET" w384] -> w336
          tunnel: w340 -> [_ w384]
          tunnel: w331 -> [w380 _]
          frame Default {
            (unwired) "%y%m%d%H%M" ("time format string (%c)")
            n153 = Format Date/Time String() -> (date/time string=w381:string)  [unwired: 3 in]
            n154 = Concatenate Strings(w381, w380) -> (→"String":string)
          }
          frame -1 {
          }
        }
        n155 = Match Pattern(string=w331, regular expression="\\[ESTOP:BAD\\]") -> (offset past match=w334:i32)  [unwired: 1 in, 3 out]
        n156 = case shown="Default" w334 {
          tunnel: w336 -> [_ w376]
          tunnel: [enum16{"cnfg", "inc", "mph", "err", "RSET"}."RSET" w376] -> w335
          frame Default {
            n157 = local write "ESTOP"(TRUE ("ESTOP")) -> ()
            n158 = local write "MPH"(0.0 ("MPH")) -> ()
          }
          frame -1 {
          }
        }
      }
      frame "Error" {
        n159 = local read "stopping"() -> (w389:bool)
        n160 = Compound Arithmetic op=OR("stop", w389, w388) -> (w391:bool)
        n161 = case shown="True" w391 {
          tunnel: [FALSE TRUE] -> w387
          frame False {
          }
          frame True {
            n162 = local write "stopping"(TRUE ("stopping")) -> ()
          }
        }
      }
    }
  }
  n163 = Tick Count (ms)() -> ()  [unwired: 1 out]
  n164 = VISA Close(VISA resource name=w10, error in (no error)=w9) -> (error out=w8:errorcluster)
  n165 = call <vilib>:"DAQmx Clear Task.vi"("task in"=w5, "error in"=w6) -> ("error out"=w4:errorcluster)  [unwired: 13 in]
  n166 = call <vilib>:"Simple Error Handler.vi"("error in (no error)"=w8) -> ()  [unwired: 4 in, 5 out]
  n167 = call <vilib>:"Simple Error Handler.vi"("error in (no error)"=w4) -> ()  [unwired: 4 in, 5 out]
  "Waveform Graph" <- dbl[] []
